vi "ADS1015_REG_CONFIG_Compiler.vi"(3 "ADS1015 Reg Config":T2, 4 "I2C_Channel_platform":T1, 5 "Error In":errorcluster, 6 "I2C Slave Address (0)":u8) -> (19 "Error Out":errorcluster)   [LabVIEW 2014]
uses:
  User Defined/I2C_Platform_Selector.ctl
  <vilib>/TSXperts/Raspberry Pi Compatible Compiler for LabVIEW/GPIO.lvlib
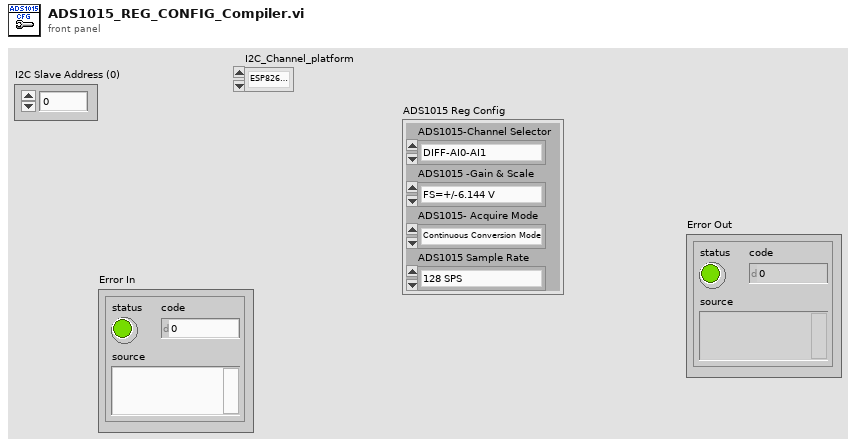
[diagram p1: front panel]
types:
  T1 = typedef "I2C_Platform_Selector.ctl" = enum16{"ESP8266-I2C", "Raspberry Pi-I2C"}
  T2 = cluster{"ADS1015-Channel Selector":enum8{"DIFF-AI0-AI1", "DIFF-AI0-AI3", "DIFF-AI1-AI3", "DIFF-AI2-AI3", "Single Ended - AI0", "Single Ended - AI1", "Single Ended - AI2", "Single Ended - AI3"}, "ADS1015 -Gain & Scale":enum8{"FS=+/-6.144 V", "FS=+/-4.096 V", "FS=+/-2.048 V", "FS=+/-1.024 V", "FS=+/-0.512 V", "FS=+/-0.256-A V", "FS=+/-0.256-B V", "FS=+/-0.256-C V"}, "ADS1015- Acquire Mode":enum16{"Continuous Conversion Mode", "Single Shot Mode"}, "ADS1015 Sample Rate":enum8{"128 SPS", "250 SPS", "490 SPS", "920 SPS", "1600 SPS", "2400 SPS", "3300 SPS", "3300 SPS A"}}
  T3 = enum8{"DIFF-AI0-AI1", "DIFF-AI0-AI3", "DIFF-AI1-AI3", "DIFF-AI2-AI3", "Single Ended - AI0", "Single Ended - AI1", "Single Ended - AI2", "Single Ended - AI3"}
  T4 = enum8{"FS=+/-6.144 V", "FS=+/-4.096 V", "FS=+/-2.048 V", "FS=+/-1.024 V", "FS=+/-0.512 V", "FS=+/-0.256-A V", "FS=+/-0.256-B V", "FS=+/-0.256-C V"}
  T5 = enum16{"Continuous Conversion Mode", "Single Shot Mode"}
  T6 = enum8{"128 SPS", "250 SPS", "490 SPS", "920 SPS", "1600 SPS", "2400 SPS", "3300 SPS", "3300 SPS A"}
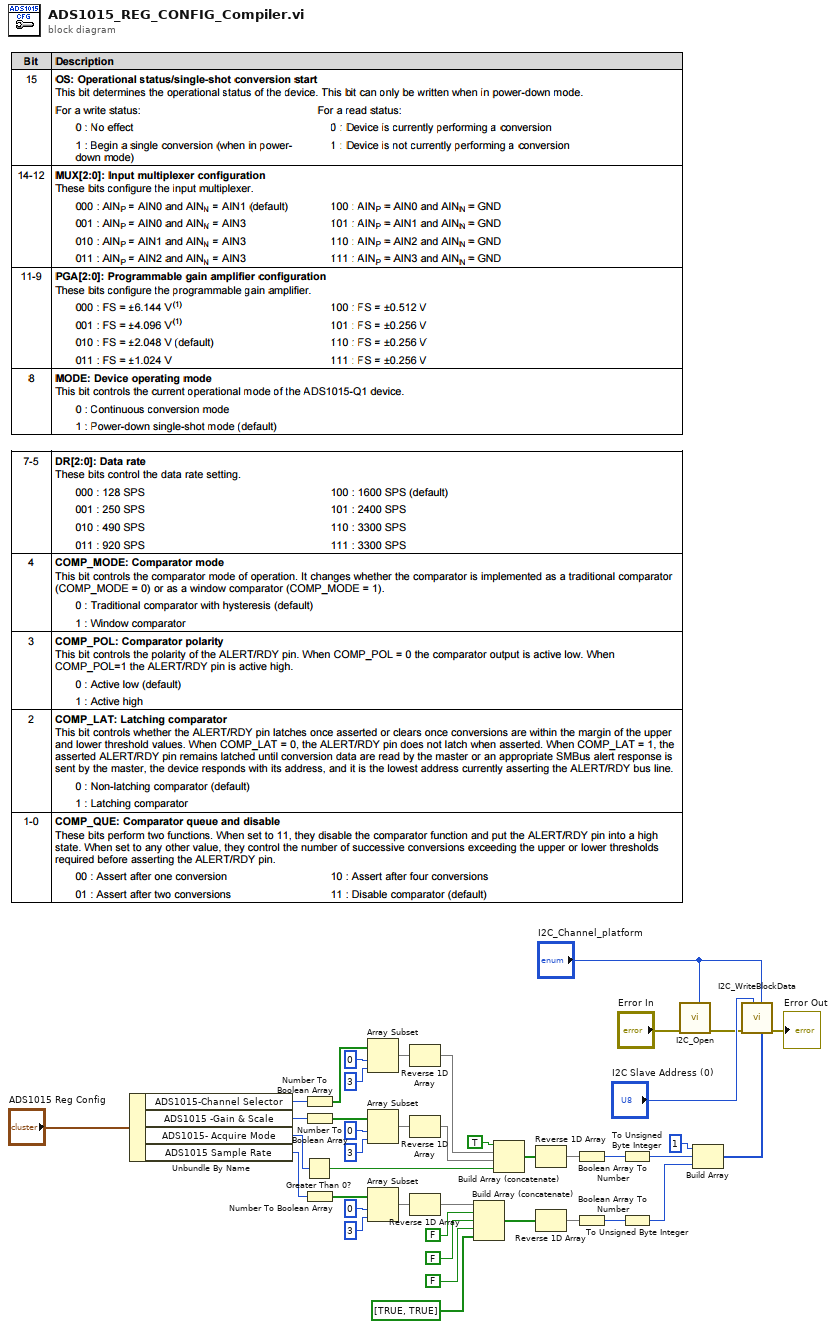
[diagram p0: block diagram]
diagram:
  n1 = Unbundle By Name("ADS1015 Reg Config") -> ("ADS1015-Channel Selector"=w10:T3, "ADS1015 -Gain & Scale"=w9:T4, "ADS1015- Acquire Mode"=w8:T5, "ADS1015 Sample Rate"=w7:T6)
  n2 = Greater Than 0?(x=w8) -> (x > 0?=w15:bool)
  n3 = Number To Boolean Array(number=w10) -> (Boolean array=w26:bool[])
  n4 = Number To Boolean Array(number=w9) -> (Boolean array=w18:bool[])
  n5 = Number To Boolean Array(number=w7) -> (Boolean array=w41:bool[])
  n6 = Array Subset(array=w26, index=0, length=3) -> (w23:bool[])
  n7 = Array Subset(array=w18, index=0, length=3) -> (w17:bool[])
  n8 = Array Subset(array=w41, index=0, length=3) -> (w38:bool[])
  n9 = Reverse 1D Array(array=w23) -> (reversed array=w21:bool[])
  n10 = Reverse 1D Array(array=w17) -> (reversed array=w16:bool[])
  n11 = Reverse 1D Array(array=w38) -> (reversed array=w37:bool[])
  n12 = Build Array (concatenate)(w37, FALSE, FALSE, FALSE, bool[] [TRUE, TRUE] ("array")) -> (w32:bool[])
  n13 = Build Array (concatenate)(TRUE, w21, w16, w15) -> (w14:bool[])
  n14 = Reverse 1D Array(array=w14) -> (reversed array=w13:bool[])
  n15 = Reverse 1D Array(array=w32) -> (reversed array=w31:bool[])
  n16 = Boolean Array To Number(Boolean array=w13) -> (number=w12:u32)
  n17 = Boolean Array To Number(Boolean array=w31) -> (number=w30:u32)
  n18 = To Unsigned Byte Integer(number=w12) -> (unsigned 8bit integer=w29:u8)
  n19 = To Unsigned Byte Integer(number=w30) -> (unsigned 8bit integer=w27:u8)
  n20 = call <vilib>:"I2C_Open.vi"("Bus"="I2C_Channel_platform", "error in"="Error In") -> ("error out"=w1:errorcluster)  [unwired: 9 in]
  n21 = Build Array(u8 1 ("element"), w29, w27) -> (w5:u8[])
  n22 = call <vilib>:"I2C_WriteBlockData.vi"("Block"=w5, "Bus"="I2C_Channel_platform", "Address"="I2C Slave Address (0)", "error in"=w1) -> ("error out"=→"Error Out":errorcluster)  [unwired: 7 in]
